vi "CLC_Power_InPhase_Cal_Channel_64.vi"(8 "error in":errorcluster, 11 "Channel IN":i32=16) -> (0 "error out":errorcluster, 1 "Channel":i32, 3 "Ref_Channel":i32)   [LabVIEW 2023]
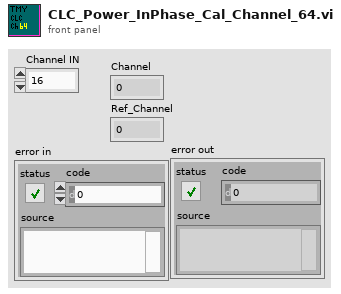
[diagram p1: front panel]
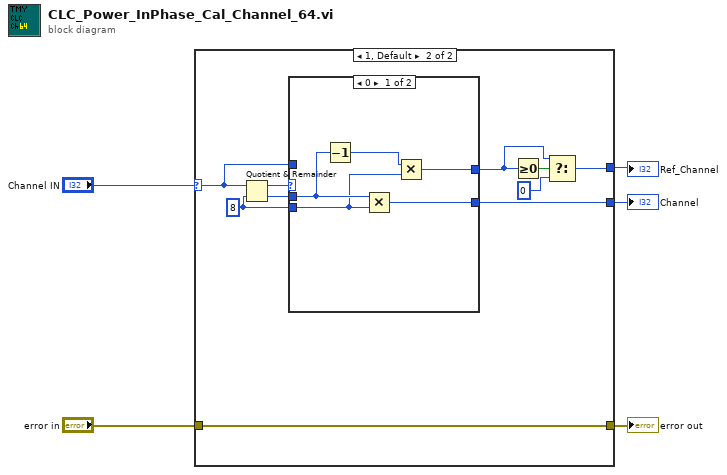
[diagram p0: block diagram]
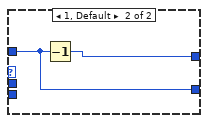
[diagram p3: hidden frame]
diagram:
  n1 = case shown="1, Default" "Channel IN" {
    selector: "Channel IN" -> [w6 w13]
    tunnel: [w6 w14] -> w4
    tunnel: [w6 w8] -> w5
    tunnel: "error in" -> [w7 w12]
    tunnel: [w7 w12] -> w1
    frame 0 {
    }
    frame 1, Default {
      w15 = 8 ("y")
      n2 = Quotient & Remainder(x=w13, y=w15) -> (x-y*floor(x/y)=w17:i32, floor(x/y)=w16:i32)
      n3 = case shown="0" w17 {
        tunnel: w16 -> [w20 _]
        tunnel: w15 -> [w19 _]
        tunnel: [w22 w24] -> w14
        tunnel: [w21 w23] -> w10
        tunnel: w13 -> [_ w24]
        frame 0 {
          n4 = Decrement(x=w20) -> (x-1=w18:i32)
          n5 = Multiply(x=w20, y=w19) -> (x*y=w22:i32)
          n6 = Multiply(x=w18, y=w19) -> (x*y=w21:i32)
        }
        frame 1, Default {
          n7 = Decrement(x=w24) -> (x-1=w23:i32)
        }
      }
      n8 = Greater Or Equal To 0?(x=w10) -> (x >= 0?=w11:bool)
      n9 = Select(t=w10, s=w11, f=0) -> (s? t:f=w8:i32)
    }
  }
  "Channel" <- w4
  "Ref_Channel" <- w5
  "error out" <- w1
